vi "test_read.vi"() -> ()   [LabVIEW 2020, in "UV-VIS_AVANTES.lvclass"]
uses:
  UV-VIS_AVANTES.lvclass
  C:/dev/TRANCON/Classes/GeneralFunctionality/GeneralFunctionality.lvclass
  C:/dev/TRANCON/Classes/Detector/Detector.lvclass
  Config/Config.lvclass
  UV-VIS_AVANTES.lvclass/UV-VIS_AVANTES.ctl
  GeneralFunctionality/GeneralFunctionality.lvclass/GeneralFunctionality.ctl
  Detector.lvclass/Detector.ctl
  Detector.lvclass
  GeneralFunctionality/GeneralFunctionality.lvclass
panel:
  out "Waveform Graph":sgl[](graph)
  in  "Path":path=path "C:/Dev/TRANCON/settings/settingsDetector.ini"
  out "error out":errorcluster
  in  "DLL path":path=path "C:/Dev/TRANCON/DLL/avaspec.dll"
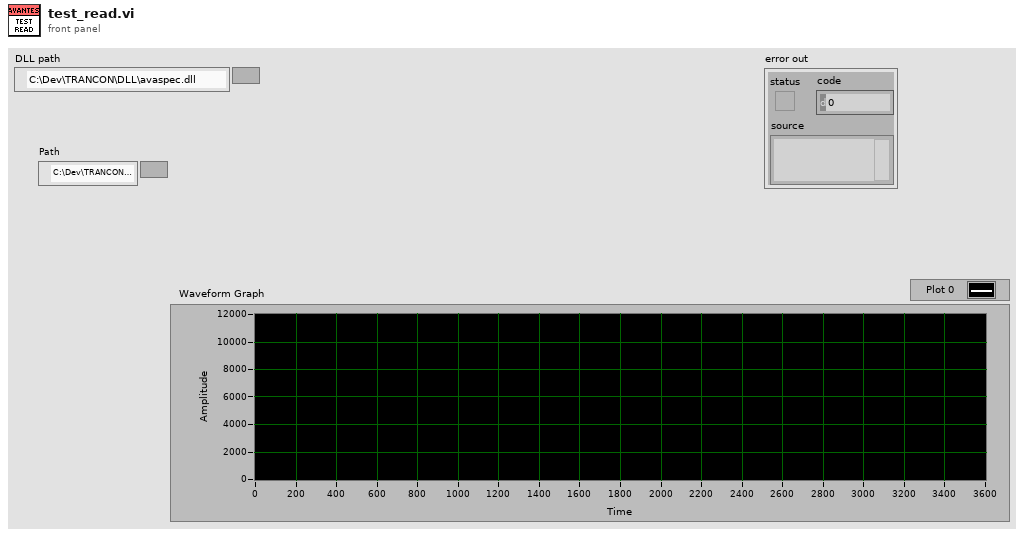
[diagram p1: front panel]
types:
  T1 = typedef "UV-VIS_AVANTES.lvclass/def_parameters.ctl" = cluster{"Len":u16, "ConfigVersion":u16, "UserFriendlyId":u8[], "DetectorType":cluster{"SensorType":u8, "NrPixels":u16, "Fit":sgl[], "NLEnable":u8, "NLCorrect":dbl[], "LowNLCounts":dbl, "HighNLCounts":dbl, "Gain":sgl[], "Reserved":sgl, "Offset":sgl[], "Extern Offset":sgl, "DefectivePixels":u16[]}, "IrradianceType":cluster{"SpectrumCalibrationType":cluster{"SmoothingType":cluster{"m_SmoothPix":u16, "SmoothModel":u8}, "CalInttime":sgl, "CalibConvers":sgl[]}, "CalibrationType":u8, "FiberDiameter":i32}, "SpectrumCalibrationType":cluster{"SmoothingType":cluster{"m_SmoothPix":u16, "SmoothModel":u8}, "CalInttime":sgl, "CalibConvers":sgl[]}, "SpectrumCorrectionType":sgl[], "StandAloneType":cluster{"StandAloneType":u8, "MeasConfigType":cluster{"StartPixel":u16, "StopPixel":u16, "IntegrationTime":sgl, "IntegrationDelay":u32, "NrAverages":u32, "DarkCorrectionType":cluster{"Enable CorDynDark":u8, "ForgetPercentage":u8}, "SmoothingType":cluster{"SmoothPix":u16, "SmoothModel":u8}, "SatDetection":u8, "TriggerType":cluster{"Trigger Mode":u8, "Trigger Source":u8, "Trigger SourceType":u8}, "ControlSettingsType":cluster{"StrobeControl":u16, "LaserDelay":u32, "LaserWidth":u32, "LaserWaveLength":sgl, "StoreToRam":u16}}, "Nmsr":i16}, "DynamicStorageType":cluster{"Nmsr":i32, "Reserved":u8[]}, "TempSensorType":sgl[], "TecControlType":cluster{"Enable":u8, "Setpoint":sgl, "Fit[NR_DAC_POL_COEF]":sgl[]}, "ProcessControlType":cluster{"AnalogLow":sgl[], "AnalogHigh":sgl[], "DigitalLow":sgl[], "DigitalHigh":sgl[]}, "EthernetSettingsType":cluster{"IpAddr":u32, "NetMask":u32, "Gateway":u32, "DhcpEnabled":u8, "TcpPort":u16, "LinkStatus":u8}, "Reserved":u8[]}
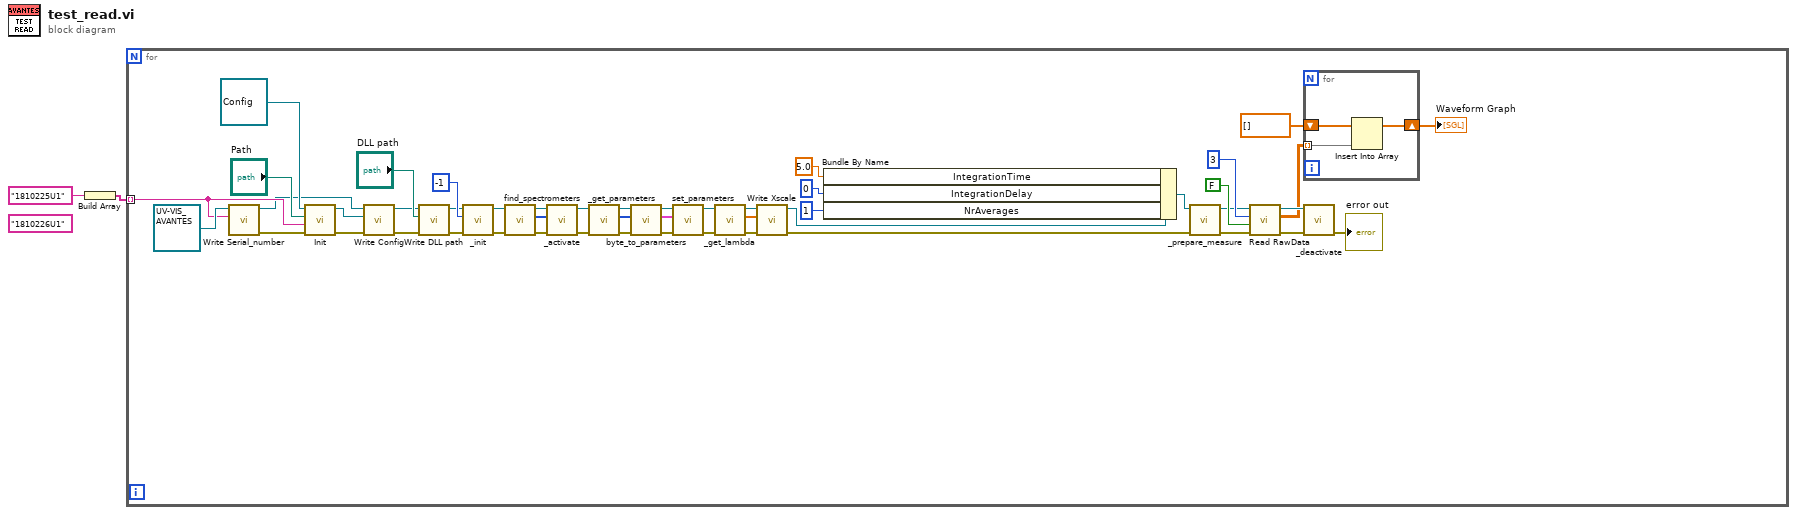
[diagram p0: block diagram]
diagram:
  (unwired) "1810226U1" ("Serial_number")
  n1 = Build Array("1810225U1" ("Serial_number")) -> (w1:string[])
  n2 = for {
    tunnel: w1 -> [w22] mode=indexing
    n3 = call "Write Serial_number.vi"("Serial_number"=w22, "UV-VIS_AVANTES in"=refnum<class "UV-VIS_AVANTES.lvclass"> refnum ("UV-VIS_AVANTES.lvclass")) -> ("error out"=w21:errorcluster, "UV-VIS_AVANTES out"=w17:refnum<class "UV-VIS_AVANTES.lvclass">)  [unwired: 8 in]
    n4 = call "Init.vi"("error in"=w21, "Name"=w22, "Path"="Path", "Config in"=refnum<class "Config.lvclass"> refnum ("Config.lvclass")) -> ("error out"=w18:errorcluster, "Config out"=w19:refnum<class "Config.lvclass">)  [unwired: 6 in]
    n5 = call "Write Config.vi"("error in (no error)"=w18, "Config.lvclass"=w19, "GeneralFunctionality en entrée"=w17) -> ("error out"=w15:errorcluster, "GeneralFunctionality en sortie"=w16:refnum<class "UV-VIS_AVANTES.lvclass">)  [unwired: 7 in]
    n6 = call "Write DLL path.vi"("error in (no error)"=w15, "DLL path"="DLL path", "Detector in"=w16) -> ("error out"=w31:errorcluster, "Detector out"=w32:refnum<class "UV-VIS_AVANTES.lvclass">)  [unwired: 7 in]
    n7 = call "_init.vi"("error in (no error)"=w31, "a_Port"=i16 -1, "UV-VIS_AVANTES in"=w32) -> ("error out"=w48:errorcluster, "UV-VIS_AVANTES out"=w49:refnum<class "UV-VIS_AVANTES.lvclass">)  [unwired: 6 in, 1 out]
    n8 = call "find_spectrometers.vi"("error in (no error)"=w48, "UV-VIS_AVANTES in"=w49) -> ("error out"=w47:errorcluster, "List Output"=w46:u8[], "UV-VIS_AVANTES out"=w50:refnum<class "UV-VIS_AVANTES.lvclass">)  [unwired: 7 in]
    n9 = call "_activate.vi"("error in (no error)"=w47, "a_pDeviceId IN"=w46, "UV-VIS_AVANTES in"=w50) -> ("error out"=w38:errorcluster, "UV-VIS_AVANTES out"=w39:refnum<class "UV-VIS_AVANTES.lvclass">)  [unwired: 7 in]
    n10 = call "_get_parameters.vi"("error in (no error)"=w38, "UV-VIS_AVANTES in"=w39) -> ("error out"=w45:errorcluster, "DeviceParam"=w44:u8[], "UV-VIS_AVANTES out"=w40:refnum<class "UV-VIS_AVANTES.lvclass">)  [unwired: 7 in]
    n11 = call "byte_to_parameters.vi"("error in (no error)"=w45, "DeviceParam"=w44, "UV-VIS_AVANTES in"=w40) -> ("error out"=w41:errorcluster, "parameters cluster"=w43:T1, "UV-VIS_AVANTES out"=w42:refnum<class "UV-VIS_AVANTES.lvclass">)  [unwired: 6 in]
    n12 = call "set_parameters.vi"("error in (no error)"=w41, "AVS_parameters"=w43, "UV-VIS_AVANTES in"=w42) -> ("error out"=w37:errorcluster, "UV-VIS_AVANTES out"=w36:refnum<class "UV-VIS_AVANTES.lvclass">)  [unwired: 7 in]
    n13 = call "_get_lambda.vi"("error in (no error)"=w37, "UV-VIS_AVANTES in"=w36) -> ("error out"=w33:errorcluster, "a_pWaveLength"=w24:dbl[], "UV-VIS_AVANTES out"=w34:refnum<class "UV-VIS_AVANTES.lvclass">)  [unwired: 7 in]
    n14 = call "Write Xscale.vi"("error in (no error)"=w33, "Xscale"=w24, "Detector en entrée"=w34) -> ("error out"=w5:errorcluster, "Detector en sortie"=w14:refnum<class "UV-VIS_AVANTES.lvclass">)  [unwired: 7 in]
    n15 = Bundle By Name(cluster=w14, "IntegrationTime"=sgl 5.0 ("parameters.StandAloneType.MeasConfigType.IntegrationTime"), "IntegrationDelay"=u32 0 ("parameters.StandAloneType.MeasConfigType.IntegrationDelay"), "NrAverages"=u32 1 ("parameters.StandAloneType.MeasConfigType.NrAverages")) -> (w6:refnum<class "UV-VIS_AVANTES.lvclass">)
    n16 = call "_prepare_measure.vi"("error in (no error)"=w5, "UV-VIS_AVANTES in"=w6) -> ("error out"=w4:errorcluster, "UV-VIS_AVANTES out"=w3:refnum<class "UV-VIS_AVANTES.lvclass">)  [unwired: 7 in, 1 out]
    n17 = call-dynamic "Read RawData.vi"("error in (no error)"=w4, "WCM_max_value"=FALSE, "# of scans"=3, "UV-VIS_AVANTES in"=w3) -> ("error out"=w12:errorcluster, "Channel I"=w10:sgl[][], "UV-VIS_AVANTES out"=w13:refnum<class "UV-VIS_AVANTES.lvclass">)  [unwired: 2 in, 3 out]
    n18 = for {
      tunnel: w10 -> [w53] mode=indexing
      shift-right: [w51] -> w8
      shift-left: sgl[] [] ("Channel I") -> [w52]
      n19 = Insert Into Array(array=w52, new element=w53) -> (w51:sgl[])  [unwired: 1 in]
    }
    "Waveform Graph" <- w8
    n20 = call "_deactivate.vi"("error in (no error)"=w12, "UV-VIS_AVANTES in"=w13) -> ("error out"=→"error out":errorcluster)  [unwired: 8 in, 1 out]
  }
